vi "Read.vi"(8 "error in (no error)":errorcluster, 11 "Input Device in":refnum<class "Input Device.lvclass">) -> (0 "error out":errorcluster, 1 "Velocity out":dbl, 2 "Direction out":cluster{dbl, dbl}, 4 "Stop?":bool, 5 "Boost?":bool)   [LabVIEW 2021, in "Input Device.lvclass"]
doc: "MIT Licence\nCopyright (c) 2024 David Grollier"
uses:
  Input Device.lvclass
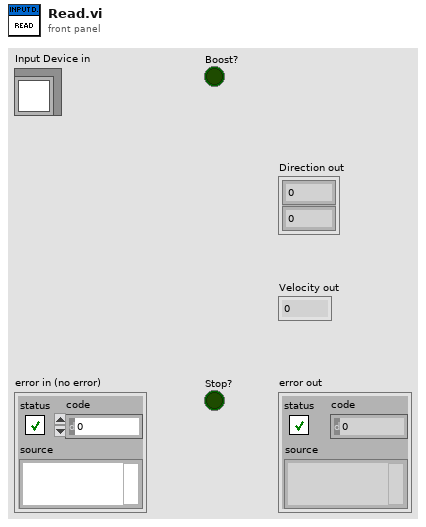
[diagram p1: front panel]
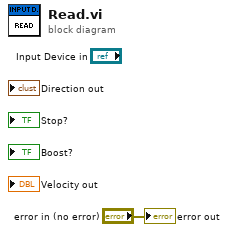
[diagram p0: block diagram]
diagram:
  "error out" <- "error in (no error)"
